vi "digital-sr-flip-flop-test.vi"() -> ()   [LabVIEW 2019]
uses:
  <vilib>/Rock Robotics/WPI/ThirdParty/JAS_Junk/TrajLib/Trajectory_Library.lvlib
panel:
  in  "Tab Control":enum32{"Control Panel", "Logic"}(tab)
  in  "Set 1":bool
  in  "Reset 1":bool
  out "Output 1":bool
  out "NOT Output 1":bool
  in  "Set 2":bool
  in  "Reset 2":bool
  out "Ouptut 2":bool
  out "NOT Output 2":bool
  out "Digital State Chart":cluster{dbl, dbl, dbl, dbl, dbl, dbl, dbl, dbl}(graph)
  # "S/R Flip-Flop Test"
  # "Set 1 and Reset 1\nHave edge on\ntriggers"
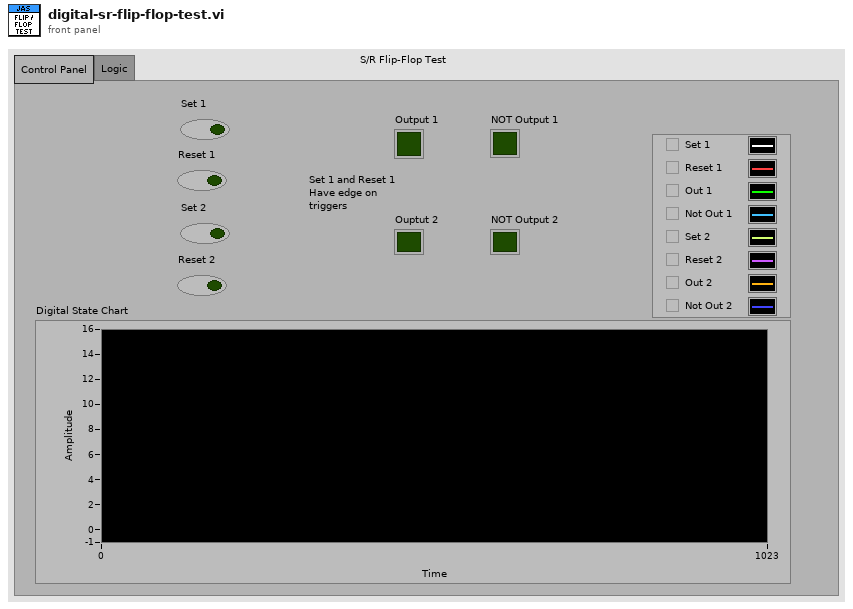
[diagram p1: front panel]
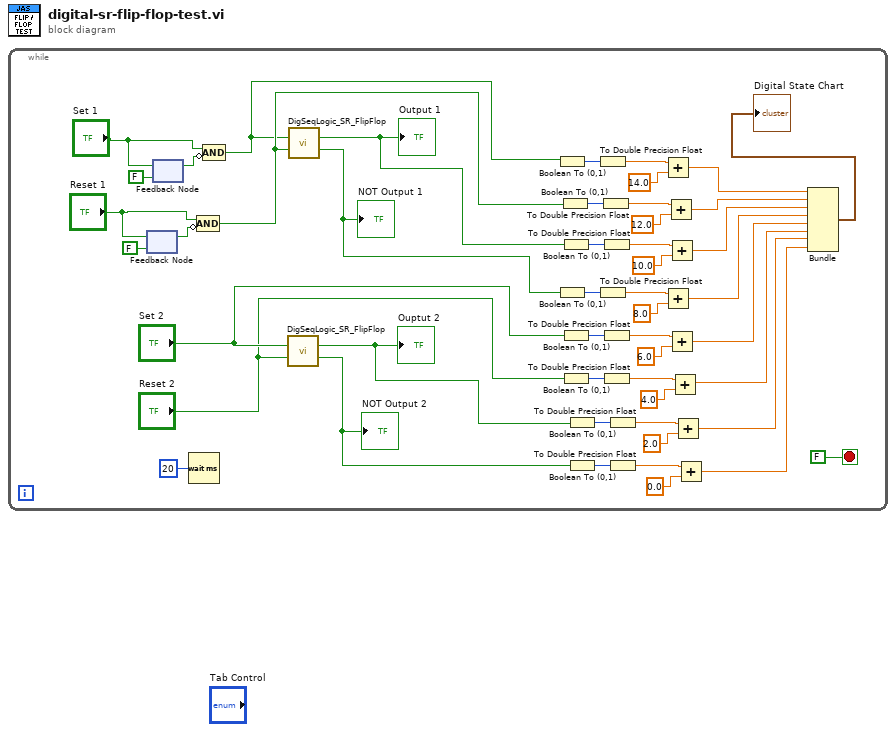
[diagram p0: block diagram]
diagram:
  n1 = while {
    stop <- FALSE stop-if-true
    n2 = feedback #1(FALSE ("Set 1")) -> (w5:bool)
    n3 = feedback-in #1("Reset 1") -> ()
    n4 = feedback-in #2("Set 1") -> ()
    n5 = feedback #2(FALSE ("Set 1")) -> (w8:bool)
    n6 = Wait (ms)(milliseconds to wait=u32 20) -> ()  [unwired: 1 out]
    n7 = Compound Arithmetic op=AND("Reset 1", invert w5) -> (w2:bool)
    n8 = Compound Arithmetic op=AND("Set 1", invert w8) -> (w1:bool)
    n9 = call <vilib>:"DigSeqLogic_SR_FlipFlop.vi"("Set"="Set 2", "Reset"="Reset 2") -> ("Output"=w10:bool, "Inverse Output"=w9:bool)  [unwired: 12 in]
    "Ouptut 2" <- w10
    "NOT Output 2" <- w9
    n10 = call <vilib>:"DigSeqLogic_SR_FlipFlop.vi"("Set"=w1, "Reset"=w2) -> ("Output"=w14:bool, "Inverse Output"=w13:bool)  [unwired: 12 in]
    "Output 1" <- w14
    "NOT Output 1" <- w13
    n11 = Boolean To (0,1)(Boolean=w1) -> (0, 1=w30:i16)
    n12 = Boolean To (0,1)(Boolean=w13) -> (0, 1=w31:i16)
    n13 = Boolean To (0,1)(Boolean=w2) -> (0, 1=w33:i16)
    n14 = Boolean To (0,1)(Boolean=w14) -> (0, 1=w35:i16)
    n15 = Boolean To (0,1)(Boolean="Set 2") -> (0, 1=w37:i16)
    n16 = Boolean To (0,1)(Boolean="Reset 2") -> (0, 1=w39:i16)
    n17 = Boolean To (0,1)(Boolean=w10) -> (0, 1=w19:i16)
    n18 = Boolean To (0,1)(Boolean=w9) -> (0, 1=w21:i16)
    n19 = To Double Precision Float(number=w30) -> (double precision float=w46:dbl)
    n20 = To Double Precision Float(number=w31) -> (double precision float=w32:dbl)
    n21 = To Double Precision Float(number=w33) -> (double precision float=w34:dbl)
    n22 = To Double Precision Float(number=w35) -> (double precision float=w36:dbl)
    n23 = To Double Precision Float(number=w37) -> (double precision float=w38:dbl)
    n24 = To Double Precision Float(number=w39) -> (double precision float=w40:dbl)
    n25 = To Double Precision Float(number=w19) -> (double precision float=w20:dbl)
    n26 = To Double Precision Float(number=w21) -> (double precision float=w22:dbl)
    n27 = Add(x=w46, y=14.0) -> (x+y=w47:dbl)
    n28 = Add(x=w32, y=8.0) -> (x+y=w45:dbl)
    n29 = Add(x=w34, y=12.0) -> (x+y=w43:dbl)
    n30 = Add(x=w36, y=10.0) -> (x+y=w44:dbl)
    n31 = Add(x=w38, y=6.0) -> (x+y=w41:dbl)
    n32 = Add(x=w40, y=4.0) -> (x+y=w42:dbl)
    n33 = Add(x=w20, y=2.0) -> (x+y=w16:dbl)
    n34 = Add(x=w22, y=0.0) -> (x+y=w15:dbl)
    n35 = Bundle(w47, w43, w44, w45, w41, w42, w16, w15) -> (→"Digital State Chart":cluster{dbl, dbl, dbl, dbl, dbl, dbl, dbl, dbl})  [unwired: 1 in]
  }
